vi "waveform to t-Y cluster (scalar).vi"(1 "waveform":waveform(dbl)) -> (0 "t-Y data":cluster{"t":dbl[], "Y":dbl[]})   [LabVIEW 2012, in "common.lvlib"]
uses:
  common.lvlib
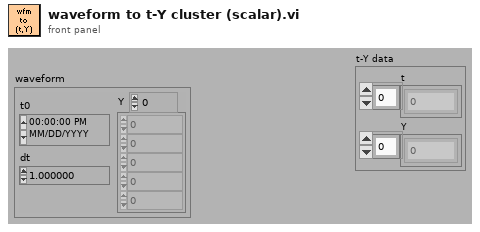
[diagram p1: front panel]
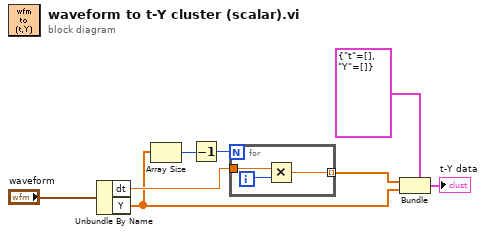
[diagram p0: block diagram]
diagram:
  n1 = Unbundle By Name("waveform") -> ("dt"=w8:dbl, "Y"=w3:dbl[])
  n2 = Array Size(array=w3) -> (size(s)=w6:i32)
  n3 = Decrement(x=w6) -> (x-1=w5:i32)
  n4 = for {
    N: w5 -> [_]
    tunnel: w8 -> [w11]
    tunnel: [w9] -> w4 mode=indexing
    i -> [w10]
    n5 = Multiply(x=w11, y=w10) -> (x*y=w9:dbl)
  }
  n6 = Bundle(cluster=cluster{"t":dbl[], "Y":dbl[]} {"t"=[], "Y"=[]} ("t-Y data"), "t"=w4, "Y"=w3) -> (→"t-Y data":cluster{"t":dbl[], "Y":dbl[]})
